vi "BasicCluster.vi"() -> ()   [LabVIEW 2016, in "test_ValueSignal.lvlib"]
uses:
  test_ValueSignal.lvlib
  Helper/HelperVI1.vi
  main/apis/Setup/GetVI/GetVIByPath.vi
  main/apis/Stimulus/ValueSignal/ValueSignalByPathString.vi
  main/apis/Assert/AssertControlValue/True.vi
  main/apis/Assert/AssertControlValue/Equal.vi
  main/Drona.lvlib
  main/apis/Stimulus/ValueSignal/ValueSignal.lvlib
  main/apis/Setup/GetVI/GetVI.lvlib
  <vilib>/addons/_JKI Toolkits/Caraya/classes/Test/Test.lvclass
  main/apis/Assert/AssertControlValue/AssertControlValue.lvlib
panel:
  out "error out":errorcluster
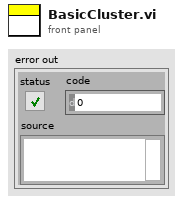
[diagram p1: front panel]
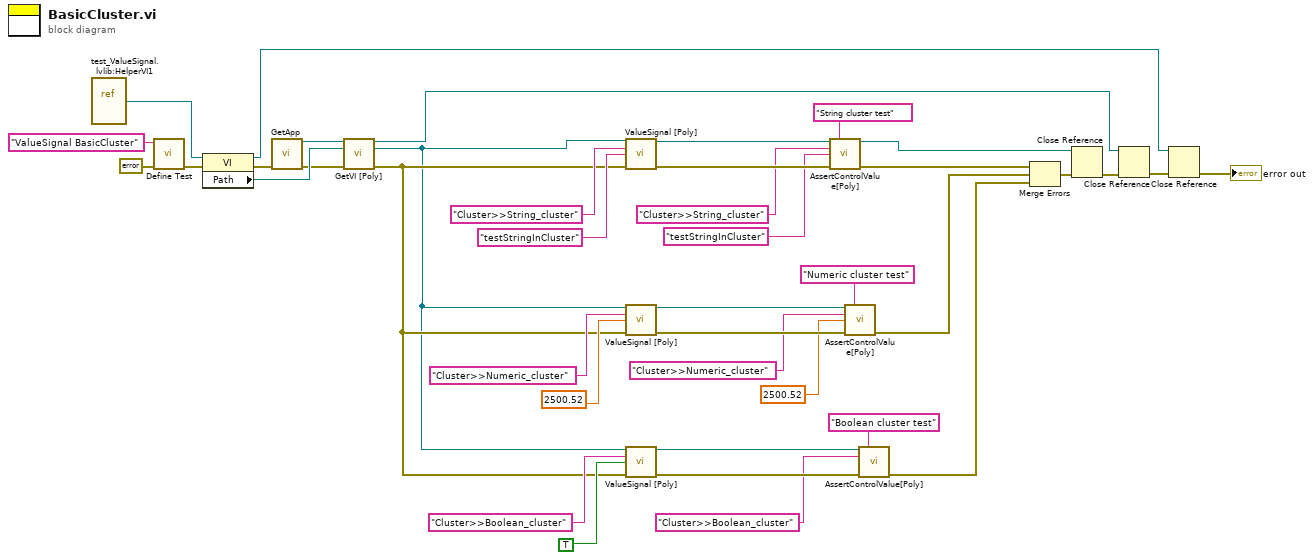
[diagram p0: block diagram]
diagram:
  n1 = vi-ref "test_ValueSignal.lvlib:HelperVI1.vi"() -> (w1:refnum<vi>)
  n2 = call <vilib>:"Define Test.vi"("error in (no error)"=errorcluster {"status"=FALSE, "code"=0, "source"=""}, "Label (VI Title)"="ValueSignal BasicCluster") -> ("error out"=w25:errorcluster)  [unwired: 9 in]
  n3 = property on="Property Node" class="VI"(reference=w1, error in=w25) -> (reference out=w20:refnum<vi>, error out=w29:errorcluster, "Path"=w28:path)
  n4 = call "GetApp.vi"("error in (no error)"=w29) -> ("Application Ref"=w30:refnum<vi>, "error out"=w27:errorcluster)  [unwired: 13 in]
  n5 = call-poly "GetVI [Poly].vi"("Application Ref in"=w30, "VI Path"=w28, "error in (no error)"=w27) -> ("Application Ref out"=w21:refnum<vi>, "VI Reference"=w22:refnum<vi>, "error out"=w23:errorcluster)  [unwired: 10 in]
  n6 = call-poly "ValueSignal [Poly].vi"("VI Reference In"=w22, "Control Name"="Cluster>>String_cluster", "Value (Signaling)"="testStringInCluster" ("Control Name"), "error in"=w23) -> ("VI Reference Out"=w17:refnum<vi>, "error out"=w19:errorcluster)  [unwired: 10 in]
  n7 = call-poly "ValueSignal [Poly].vi"("VI Reference In"=w22, "Control Name"="Cluster>>Numeric_cluster", "Value (Signaling)"=2500.52, "error in"=w23) -> ("VI Reference Out"=w10:refnum<vi>, "error out"=w12:errorcluster)  [unwired: 10 in]
  n8 = call-poly "ValueSignal [Poly].vi"("VI Reference In"=w22, "Control Name"="Cluster>>Boolean_cluster", "Value (Signaling)"=TRUE, "error in"=w23) -> ("VI Reference Out"=w3:refnum<vi>, "error out"=w6:errorcluster)  [unwired: 10 in]
  n9 = call-poly "AssertControlValue[Poly].vi"("VI Reference In"=w17, "Label"="String cluster test" ("Label (VI Title)"), "Control Name"="Cluster>>String_cluster", "Control Value"="testStringInCluster" ("Control Name"), "Error In"=w19) -> ("VI Reference Out"=w14:refnum<vi>, "Error Out"=w18:errorcluster)  [unwired: 9 in]
  n10 = call-poly "AssertControlValue[Poly].vi"("VI Reference In"=w10, "Label"="Numeric cluster test" ("Label (VI Title)"), "Control Name"="Cluster>>Numeric_cluster", "Control Value"=2500.52, "Error In"=w12) -> ("Error Out"=w11:errorcluster)  [unwired: 9 in, 1 out]
  n11 = call-poly "AssertControlValue[Poly].vi"("VI Reference In"=w3, "Label"="Boolean cluster test" ("Label (VI Title)"), "Control Name"="Cluster>>Boolean_cluster", "Error In"=w6) -> ("Error Out"=w5:errorcluster)  [unwired: 10 in, 1 out]
  n12 = Merge Errors(w18, w11, w5) -> (w35:errorcluster)
  n13 = Close Reference(reference=w14, error in (no error)=w35) -> (error out=w38:errorcluster)
  n14 = Close Reference(reference=w21, error in (no error)=w38) -> (error out=w37:errorcluster)
  n15 = Close Reference(reference=w20, error in (no error)=w37) -> (error out=→"error out":errorcluster)
